vi "Source Fetch query.vi"(8 "error in (no error)":errorcluster, 11 "VISA resource name":refnum<visa-resource-name>) -> (0 "error out":errorcluster, 2 "Result":string, 3 "VISA resource name out":refnum<visa-resource-name>)   [LabVIEW 2025, in "Chroma 19052.lvlib"]
doc: "Chroma\n5 Clock Tower Place Suite 210\nMaynard, MA 01754\nTel: 1 800 253-1230\nTel: 1 877 4 A HIPOT\nFax: 1 978-461-4295\nWebsite: www.chroma.com"
uses:
  <instrlib>/Chroma 19052/Chroma 19052.lvlib
panel:
  # "FETCH?"
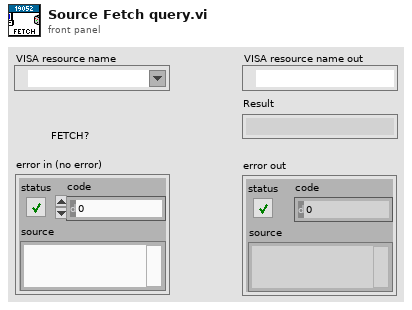
[diagram p1: front panel]
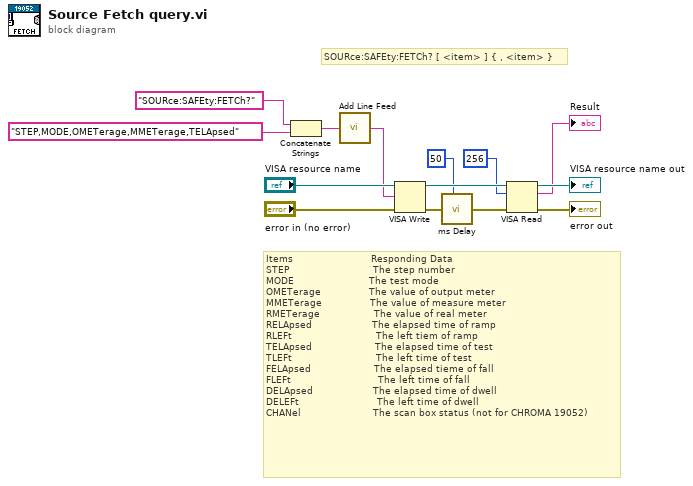
[diagram p0: block diagram]
diagram:
  # "SOURce:SAFEty:FETCh? [ <item> ] { , <item> }"
  # "Items                          Responding Data\nSTEP                            The step number\nMODE                         The test mode\nOMETerage                The value of output meter\nMMETerage                The value of measure meter\nRMETerage                  The value of real meter\nRELApsed                    The elapsed time of ramp \nRLEFt                            The left tiem of ramp\nTELApsed                     The elapsed time of test\nTLEFt                            The left time of test\nFELApsed                     The elapsed tieme of fall\nFLEFt                             The left time of fall\nDELApsed                    The elapsed time of dwell\nDELEFt                          The left time of dwell\nCHANel                        The scan box status (not for CHROMA 19052)"
  n1 = Concatenate Strings("SOURce:SAFEty:FETCh?", "STEP,MODE,OMETerage,MMETerage,TELApsed") -> (w7:string)
  n2 = call <instrlib>:"Add Line Feed.vi"("Command string"=w7) -> ("Concatenated string"=w12:string)  [unwired: 4 in]
  n3 = VISA Write(VISA resource name="VISA resource name", write buffer=w12, error in (no error)="error in (no error)") -> (VISA resource name out=w6:refnum<visa-resource-name>, error out=w2:errorcluster)  [unwired: 1 out]
  n4 = call <instrlib>:"ms Delay.vi"("miliseconds to wait"=u32 50 ("Time Delay ms"), "error in (no error)"=w2) -> ("error out"=w3:errorcluster)  [unwired: 6 in, 1 out]
  n5 = VISA Read(VISA resource name=w6, byte count=u32 256, error in (no error)=w3) -> (VISA resource name out=→"VISA resource name out":refnum<visa-resource-name>, read buffer=→"Result":string, error out=→"error out":errorcluster)  [unwired: 1 out]
